vi "Do Evaluate Fitness.vi"(8 "error in":errorcluster, 10 "IChromosome in":refnum<class "IChromosome.lvclass">, 11 "Fitness Agent in":refnum<class "Fitness Agent.lvclass">) -> (0 "error out":errorcluster, 2 "IChromosome out":refnum<class "IChromosome.lvclass">, 3 "Fitness Agent out":refnum<class "Fitness Agent.lvclass">)   [LabVIEW 2016, in "Fitness Agent.lvclass"]
uses:
  Fitness Agent.lvclass
  IChromosome/IChromosome.lvclass
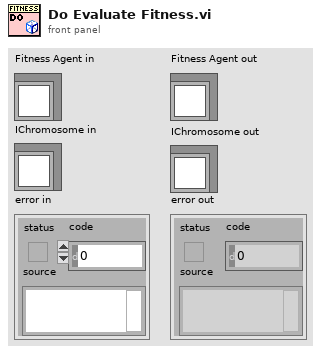
[diagram p1: front panel]
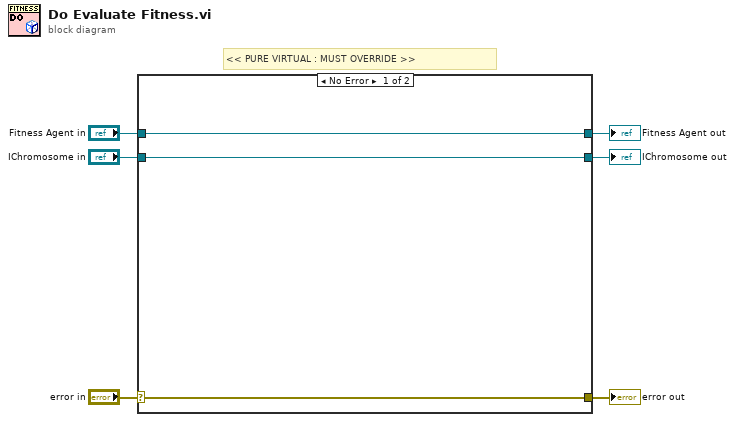
[diagram p0: block diagram]
diagram:
  # "<< PURE VIRTUAL : MUST OVERRIDE >>"
  n1 = case shown="No Error" "error in" {
    selector: "error in" -> [w8 w12]
    tunnel: [w8 w12] -> w5
    tunnel: [w9 w11] -> w3
    tunnel: "Fitness Agent in" -> [w9 w11]
    tunnel: "IChromosome in" -> [w7 w10]
    tunnel: [w7 w10] -> w1
    frame No Error {
    }
    frame Error {
    }
  }
  "error out" <- w5
  "Fitness Agent out" <- w3
  "IChromosome out" <- w1
